vi "get voltage range byte.vi"(8 "error in (no error)":errorcluster caption="에러 입력(에러 없음)", 10 "voltage range":dbl, 11 "DW7800 입력":refnum<class "DW7800.lvclass">) -> (0 "error out":errorcluster caption="에러 출력", 2 "byte value":u8 format="%02x", 3 "DW7800 출력":refnum<class "DW7800.lvclass">)   [LabVIEW 2020, in "DW7800.lvclass"]
uses:
  DW7800.lvclass
  adf26084-f599-4f22-a855-04d1fe8782d4.vi
  <vilib>/Comparison/Equal/Equal Functor/Equal Functor.lvclass
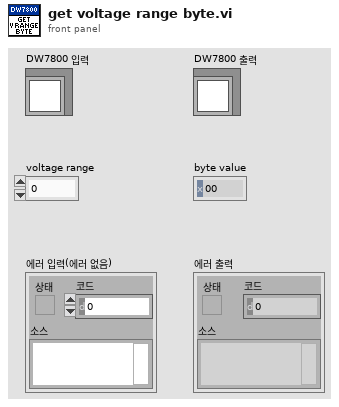
[diagram p1: front panel]
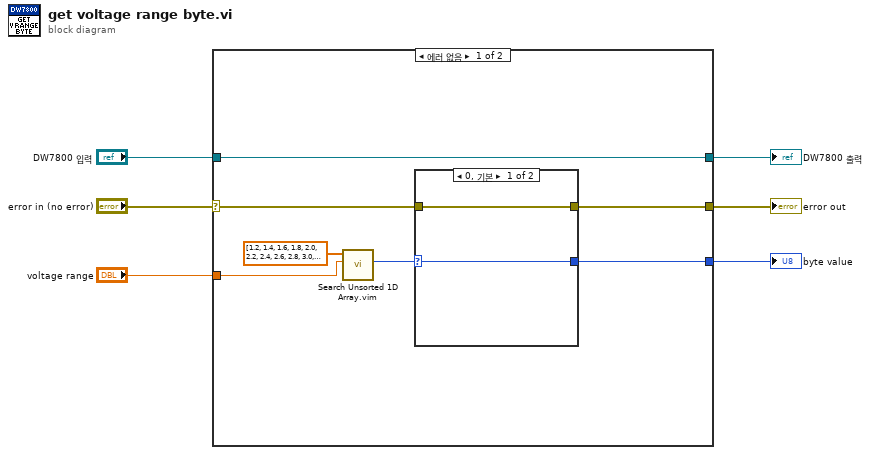
[diagram p0: block diagram]
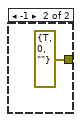
[diagram p2: hidden frame]
diagram:
  n1 = case shown="에러 없음" "error in (no error)" {
    selector: "error in (no error)" -> [w10 w18]
    tunnel: [w7 w18] -> w3
    tunnel: "DW7800 입력" -> [w13 w17]
    tunnel: [w13 w17] -> w5
    tunnel: "voltage range" -> [w11 _]
    tunnel: [w8 _] -> w1
    frame No Error {
      n2 = call "Search Unsorted 1D Array.vim"("element"=w11, "unsorted 1D array"=dbl[] [1.2, 1.4, 1.6, 1.8, 2.0, 2.2, 2.4, 2.6, 2.8, 3.0, 3.2, 3.4, 3.6]) -> ("index of element"=w9:i32)  [unwired: 9 in]
      n3 = case shown="0, 기본" w9 {
        selector: w9 -> [w15 _]
        tunnel: w10 -> [w14 _]
        tunnel: [w15 _] -> w8
        tunnel: [w14 errorcluster {"status"=TRUE, "code"=0, "source"=""} ("error IO")] -> w7
        frame 0, Default {
        }
        frame -1 {
        }
      }
    }
    frame Error {
    }
  }
  "error out" <- w3
  "DW7800 출력" <- w5
  "byte value" <- w1
